vi "fa v2.vi"(7 "fbeta":dbl, 9 "Constants and System Parameters":T1, 10 "Ankle Angle":dbl) -> (2 "fa":dbl)   [LabVIEW 2018]
uses:
  Constants and System Parameters.ctl
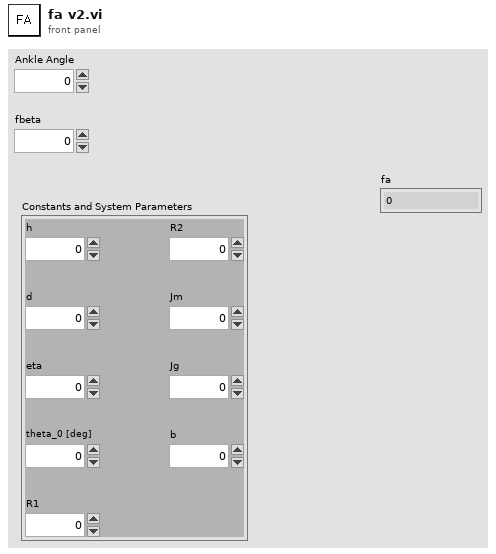
[diagram p1: front panel]
types:
  T1 = typedef "Constants and System Parameters.ctl" = cluster{"h":dbl, "d":dbl, "eta":dbl, "theta_0 [deg]":dbl, "R1":dbl, "R2":dbl, "Jm":dbl, "Jg":dbl, "b":dbl}
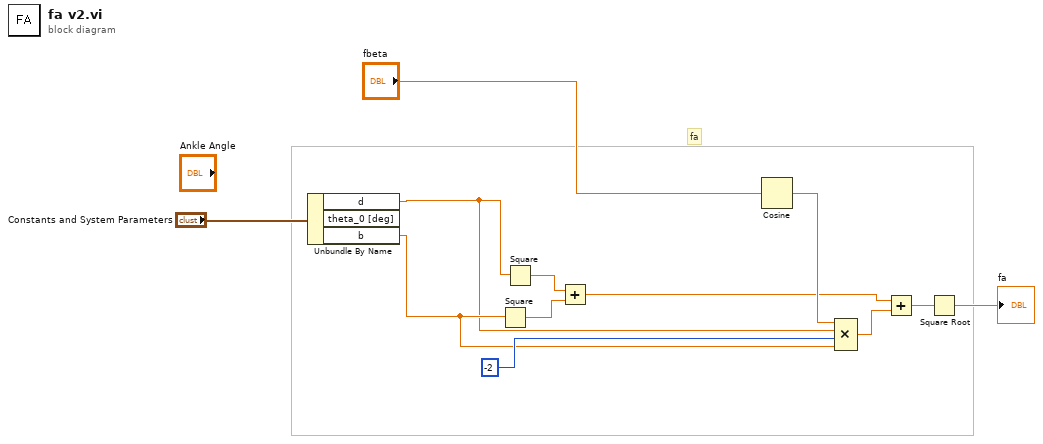
[diagram p0: block diagram]
diagram:
  # "fa"
  n1 = Unbundle By Name("Constants and System Parameters") -> ("d"=w8:dbl, "b"=w9:dbl)  [unwired: 1 out]
  n2 = Square(x=w9) -> (x^2=w11:dbl)
  n3 = Square(x=w8) -> (x^2=w12:dbl)
  n4 = Add(x=w12, y=w11) -> (x+y=w6:dbl)
  n5 = Cosine(x="fbeta") -> (cos(x)=w7:dbl)
  n6 = Compound Arithmetic op=MULTIPLY(w7, w8, -2, w9) -> (w5:dbl)
  n7 = Add(x=w6, y=w5) -> (x+y=w4:dbl)
  n8 = Square Root(x=w4) -> (sqrt(x)=→"fa":dbl)
